vi "Sonicator Module (Main).vi"(7 "Name of Parent Panel":string="Main.vi", 9 "New Center Coords":T1={"Horizontal"=470, "Vertical"=200}, 10 "Config":variant, 11 "Main UI Message Queue":refnum<queue>) -> ()   [LabVIEW 2018, in "Sonicator Module.lvlib"]
doc: "This Continuous Measurement sample project is based on the Queued Message Handler template.\n\nThe Event Handling Loop generates messages based on user interface actions.\n\nThe Message Handling Loop processes messages generated by the Event Handling Loop, or by other messages. There are also Acquisition and Logging message handling loop subVIs, and a chart updating loop."
uses:
  Sonicator Module.lvlib
  support/Message Queue/Message Cluster.ctl
  <vilib>/Utility/miscctls.llb/LVPoint32TypeDef.ctl
  controls/UI State.ctl
  Feed Module/Controls/Sonicator Module Config Cluster.ctl
  Feed Module/Controls/Sonicator Module Settings Cluster.ctl
  Sonic Systems P100/Sonic Systems P100 Settings.ctl
  Feed Module/Controls/Sonicator Module State Cluster.ctl
  Pump Module Folder/Measure Instrument/State Enum.ctl
  Sequencing/Squence Update Cluster.ctl
  Measure Instrument/State Enum.ctl
  Feed Module/Controls/Sonicator Module Display.ctl
  support/Message Queue/Enqueue Message (Single).vi
  support/User Event - Stop/User Event - Stop.lvlib
  support/Message Queue/Message Queue.lvlib
  support/Support Library.lvlib
  Measure Instrument/Sonicator Module Engine.lvlib
  Sonicator Settings Dialog.vi
  support/Command Log VIs/Command Logging.lvlib
  Sonic Systems P100/Sonic Systems P100.lvlib
  Pump Module Folder/Measure Instrument/Pump Module Engine.lvlib
  Sequencing/Sequencing Library.lvlib
  Measure Instrument/Feed Module Engine.lvlib
  Report Generation/Report Generation.lvlib
panel:
  in  "Settings Button":bool
  out "Display Cluster":cluster{"User Name":string, "µm":dbl, "W":dbl} {"W" format="%#_5f"; "µm" format="%#_5f"}
  out "Ring":u16(ring)=2
  out "Original Width":u32
  out "Original Height":u32
  out "H/W":dbl
  out "ScanCode":i16
  out "Log File path":path
  out "Status":string
  in  "Exit":bool
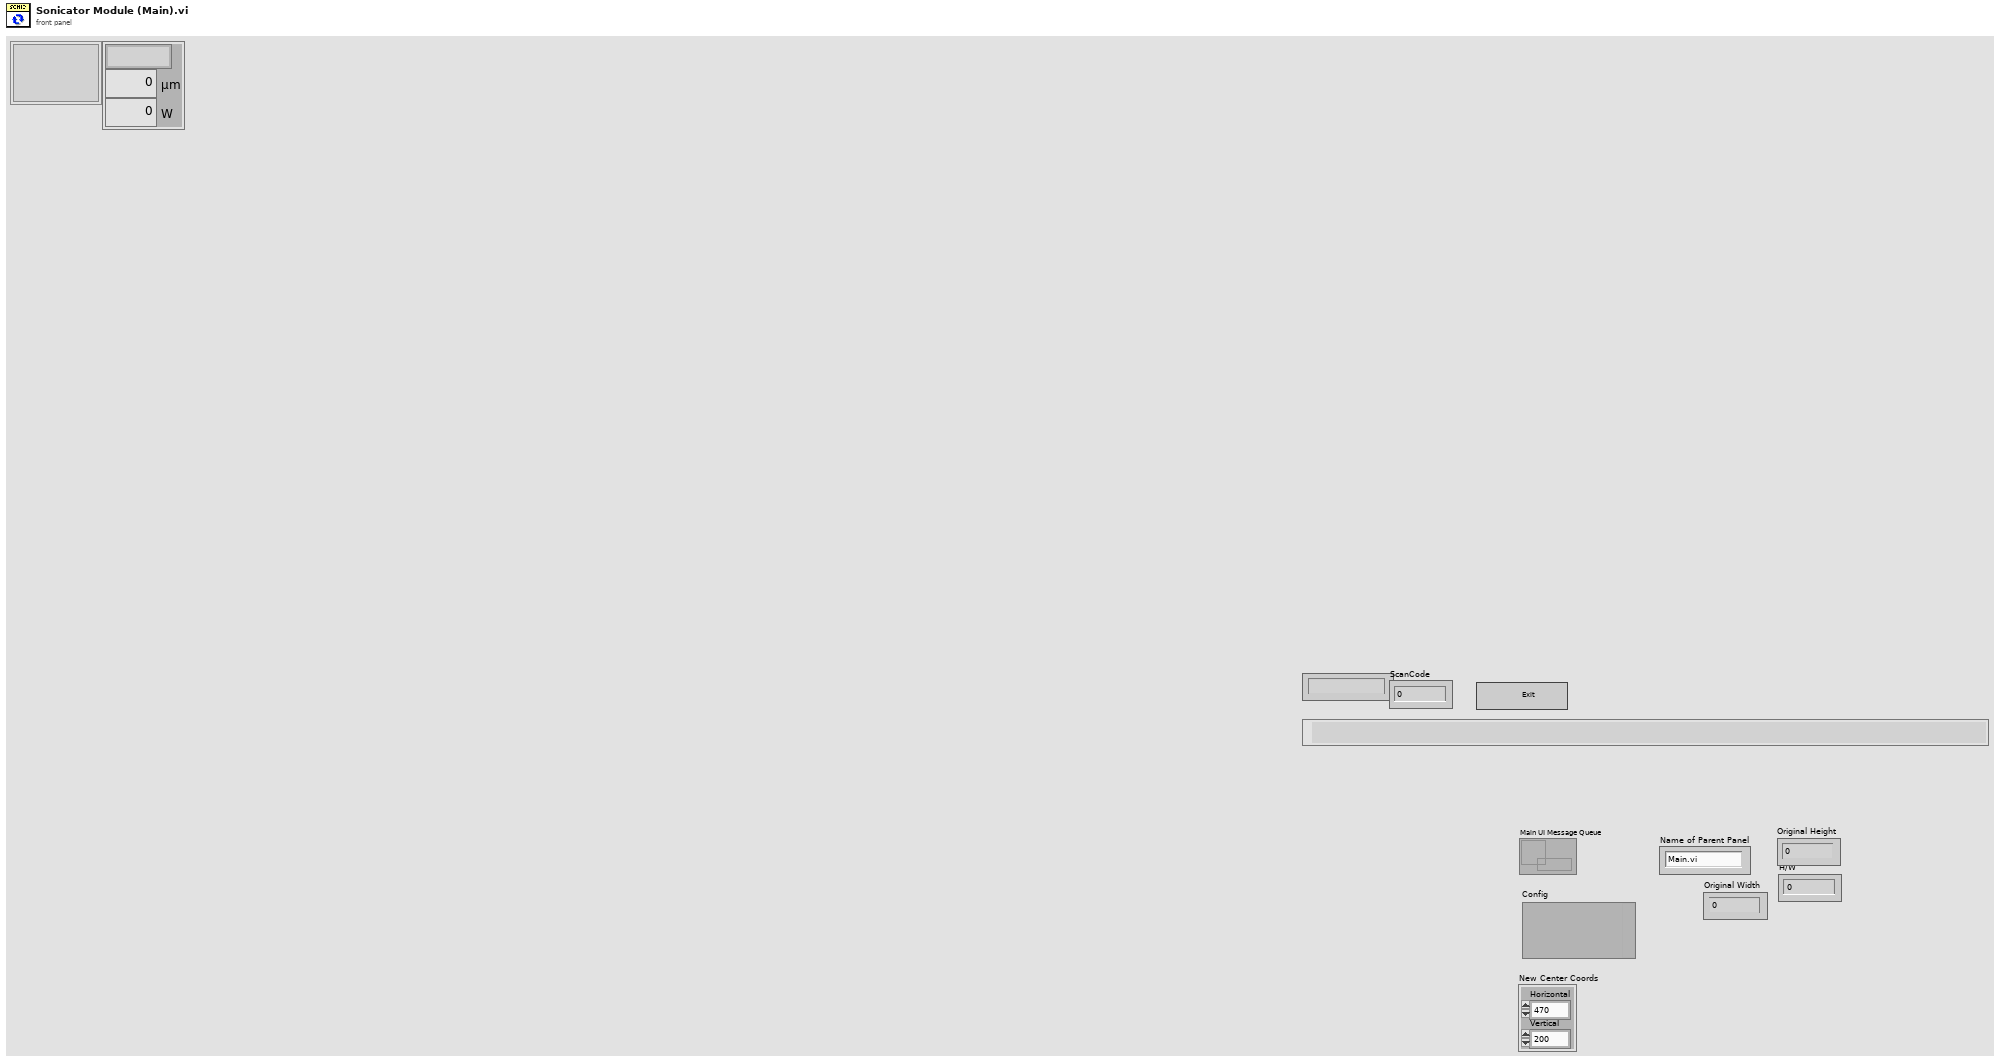
[diagram p1: front panel]
types:
  T1 = typedef "LVPoint32TypeDef.ctl" = cluster{"Horizontal":i32, "Vertical":i32}
  T2 = enum32{"Invalid", "Default", "Floating", "Floating/Auto-Hide", "Modal"}
  T3 = typedef "Sonicator Module.lvlib/Sonicator Module Config Cluster.ctl" = cluster{"GUID":string, "Drop Coords":T1, "Process Name":string, "User name":string, "Queue Name":string, "Settings":T4, "Load Count":i32}
  T4 = typedef "Sonicator Module.lvlib/Sonicator Module Settings Cluster.ctl" = cluster{"Cycle Period":dbl, "Sonicator Type":string, "SS P100 Settings":T5, "Setpoint (µm)":dbl, "Cutoff (W)":dbl}
  T5 = typedef "Sonic Systems P100.lvlib/Sonic Systems P100 Settings.ctl" = cluster{"VISA resource name":refnum<visa-resource-name>, "Simulated?":bool}
  T6 = typedef "UI State.ctl" = enum16{"Idle", "Acquiring and Logging", "Waiting for Exit", "Waiting for Exit (Acq Stopped)", "Waiting for Exit (Log Stopped)", "Waiting for Stop", "Waiting for Stop (Acq Stopped)", "Waiting for Stop (Log Stopped)"}
  T7 = typedef "Sonicator Module.lvlib/Sonicator Module State Cluster.ctl" = cluster{"State":T8, "Start Time":timestamp, "Current Time":timestamp, "Sonicator Module Config":T3, "Output Error":bool, "Log Started":bool, "First Iteration":bool, "Data":cluster{"Sonicator Amp Value":dbl, "Sonicator Power Value":dbl}, "Sonicator On?":enum16{"Off", "On", "Not Initialized", "Over Cutoff"}}
  T8 = typedef "Pump Module.lvlib/Pump Module Engine.lvlib/State Enum.ctl" = enum16{"Measuring", "Idle", "Paused"}
  T9 = typedef "LVPointTypeDef.ctl" = cluster{"Horizontal":i16, "Vertical":i16}
  T10 = typedef "Sonicator Module.lvlib/Sonicator Message Queues.ctl" = cluster{"Sonicator UI":refnum<queue>, "Sonicator Engine":refnum<queue>, "Sonicator Display":refnum<queue>}
  T11 = typedef "Sequencing Library.lvlib/Squence Update Cluster.ctl" = cluster{"Auto?":bool, "Manual Entry":dbl, "Setpoint":dbl}
  T12 = typedef "Feed Module.lvlib/Feed Module Engine.lvlib/State Enum.ctl" = enum16{"Measuring", "Idle", "Paused"}
  T13 = typedef "Sonicator Module.lvlib/Sonicator Module Display.ctl" = cluster{"Sonicator On?":enum16{"Off", "On", "Not Initialized", "Over Cutoff"}, "Sonicator Amp Value":dbl, "Sonicator Power Value":dbl, "Cycle Period":dbl}
  T14 = enum16{"Off", "On", "Not Initialized", "Over Cutoff"}
  T15 = typedef "LVRectTypeDef.ctl" = cluster{"Left":i16, "Top":i16, "Right":i16, "Bottom":i16}
  T16 = cluster{"Shift":bool, "Ctrl":bool, "Alt":bool, "Cmd":bool, "Opt":bool}
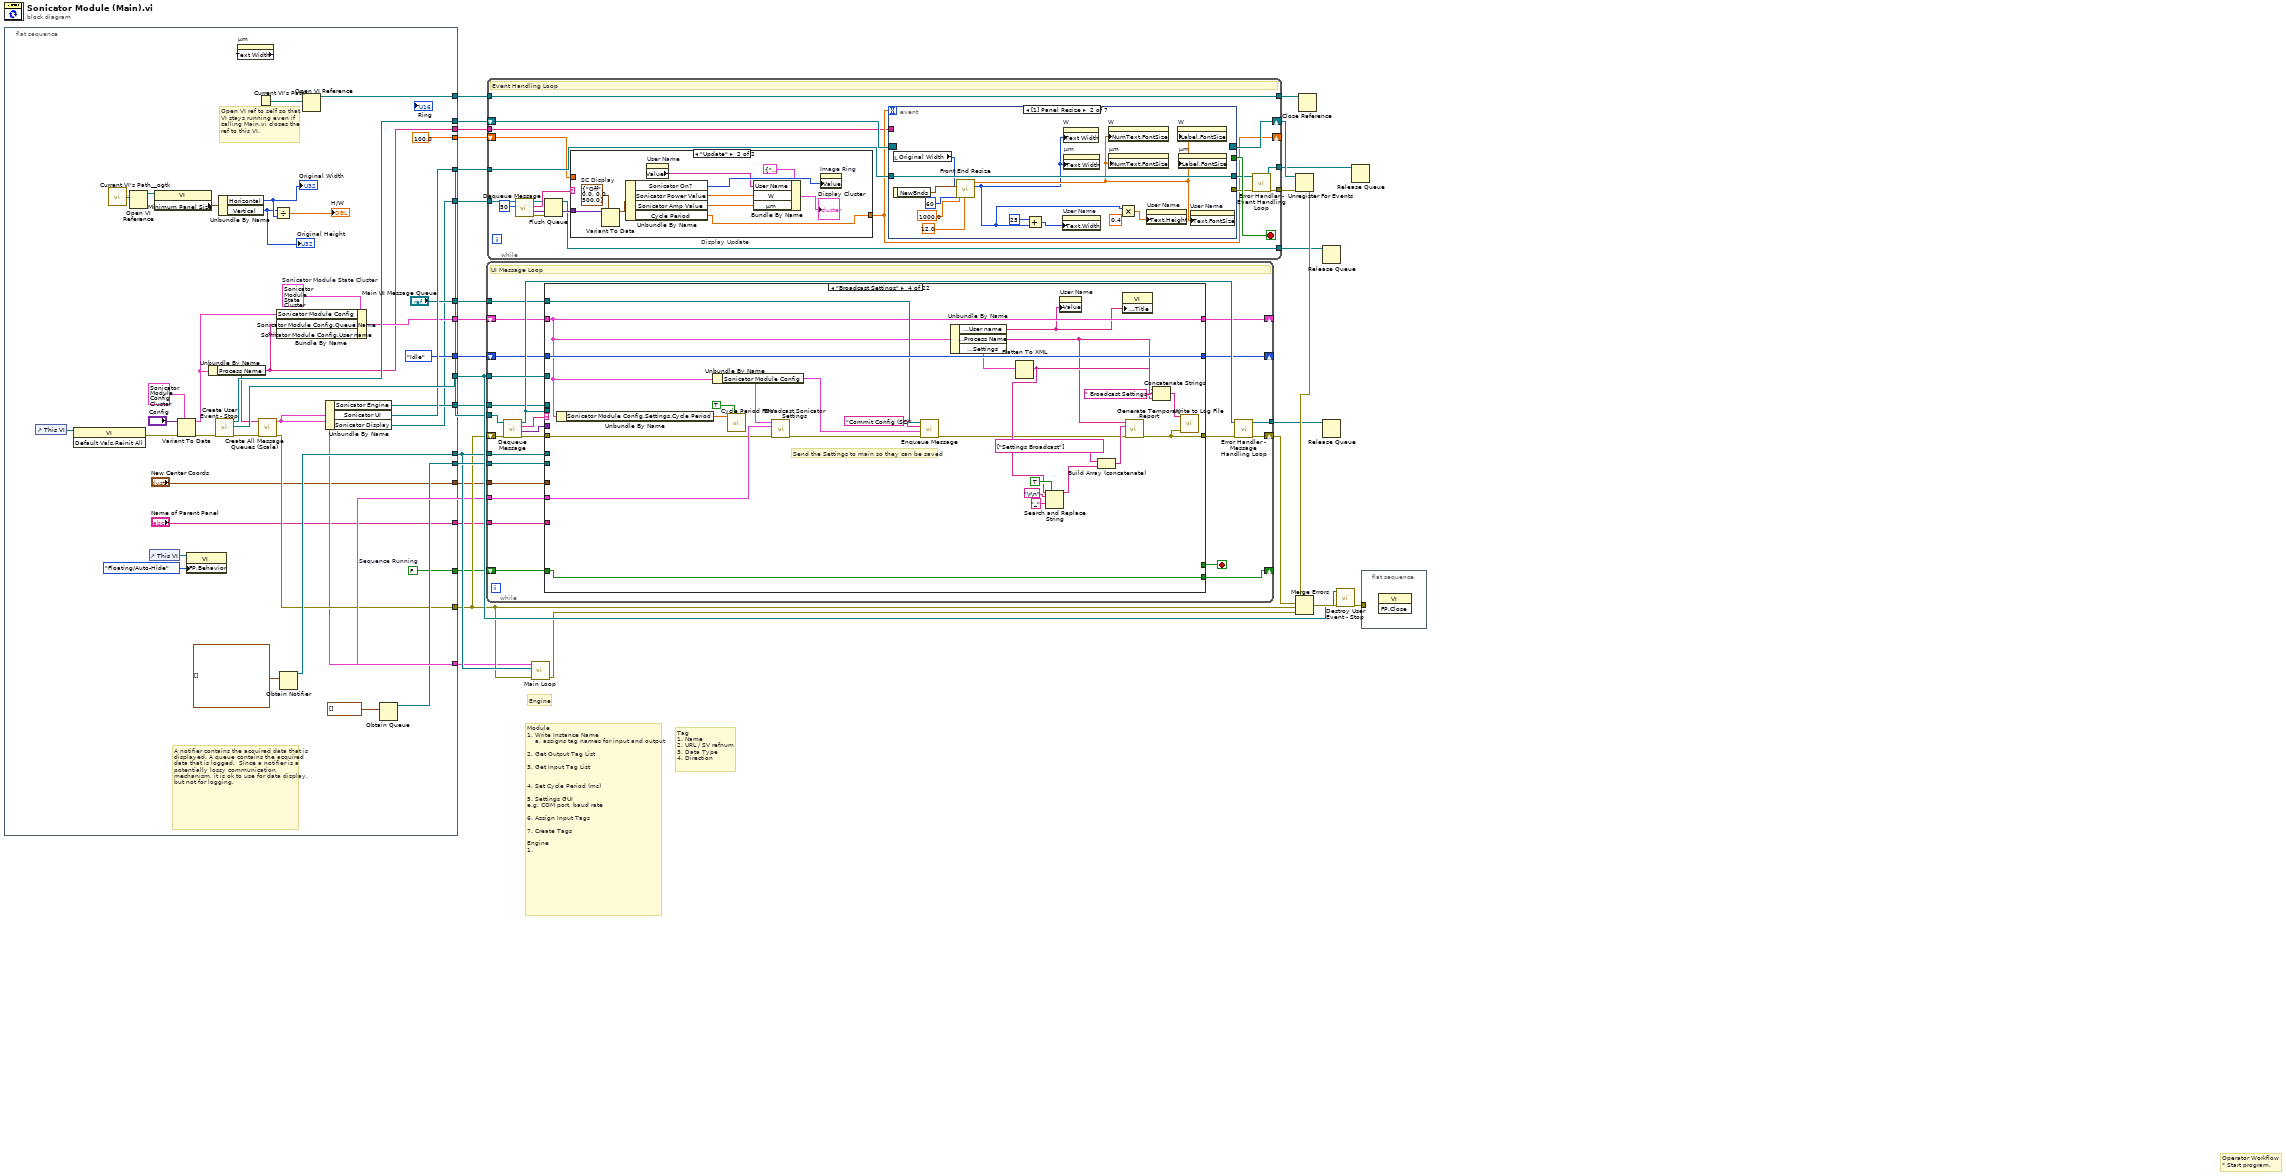
[diagram p0: block diagram]
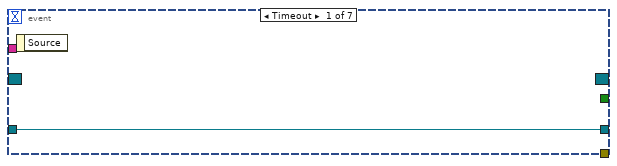
[diagram p3: hidden frame]
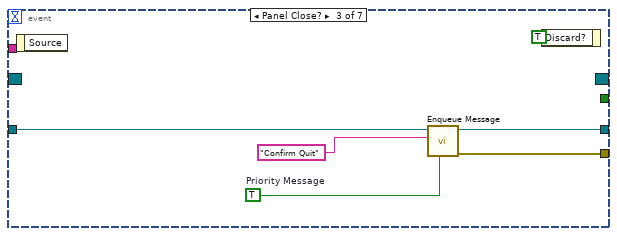
[diagram p4: hidden frame]
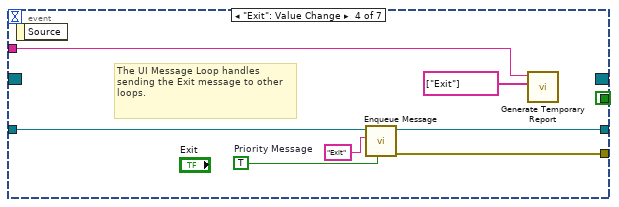
[diagram p5: hidden frame]
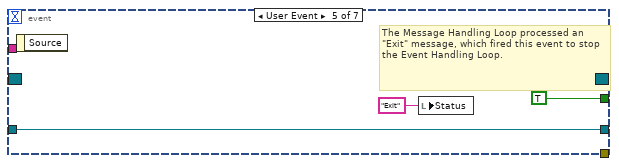
[diagram p6: hidden frame]
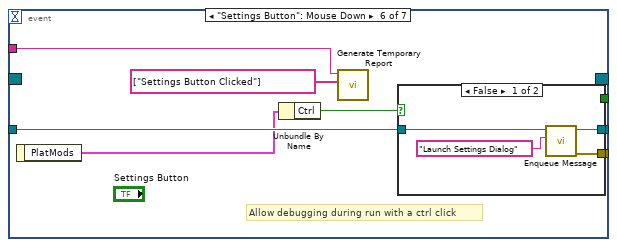
[diagram p7: hidden frame]
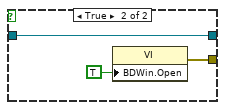
[diagram p8: hidden frame]
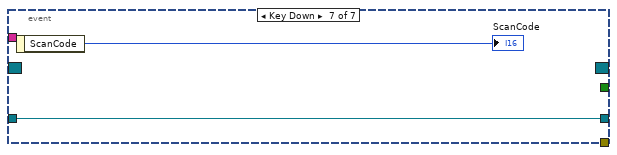
[diagram p9: hidden frame]
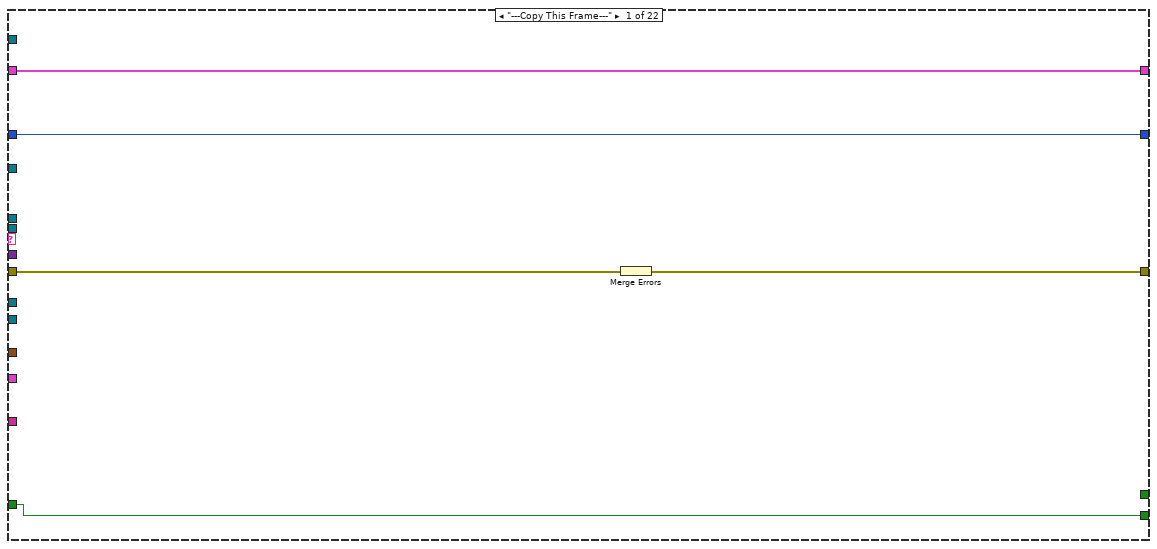
[diagram p10: hidden frame]
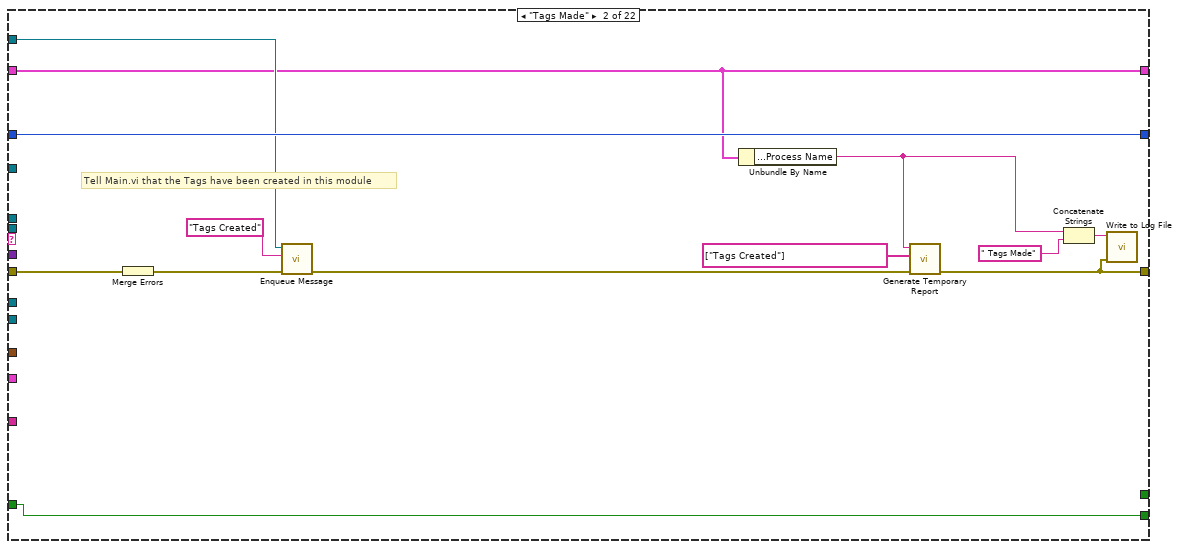
[diagram p11: hidden frame]
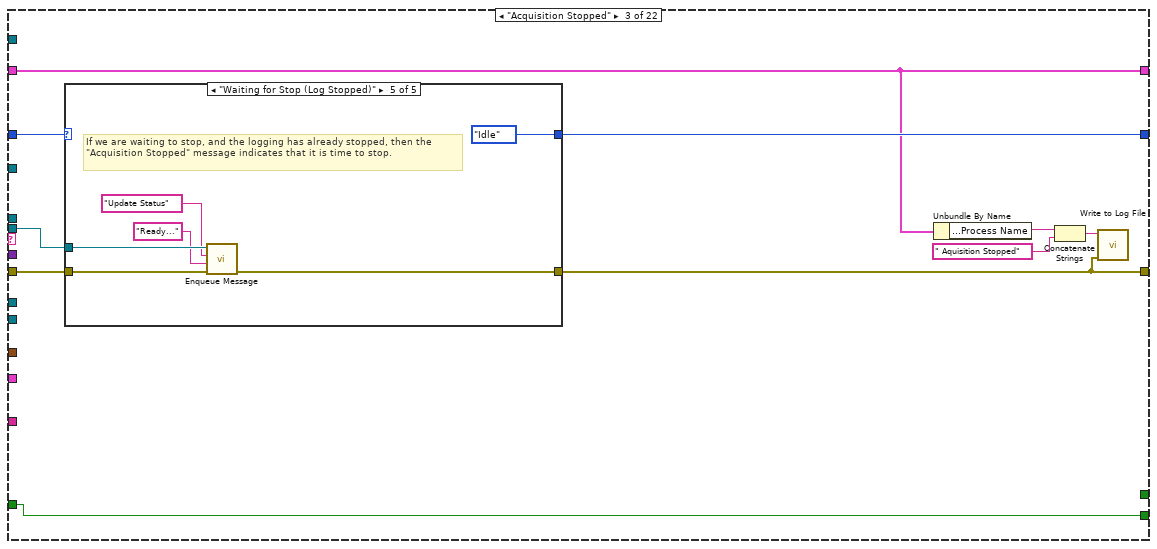
[diagram p12: hidden frame]
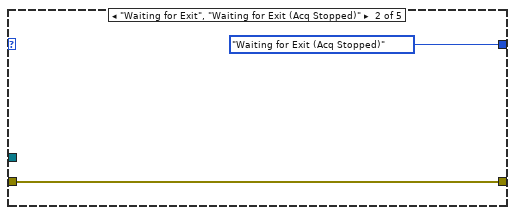
[diagram p14: hidden frame]
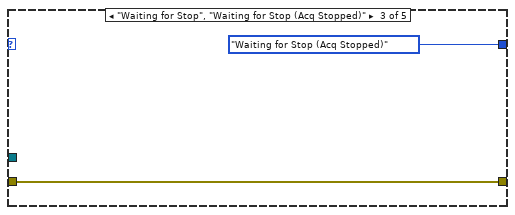
[diagram p15: hidden frame]
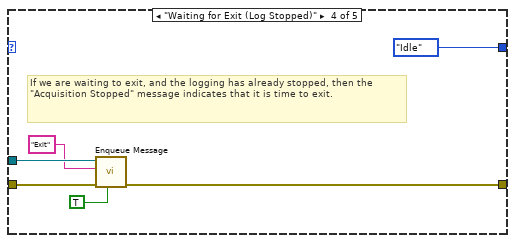
[diagram p16: hidden frame]
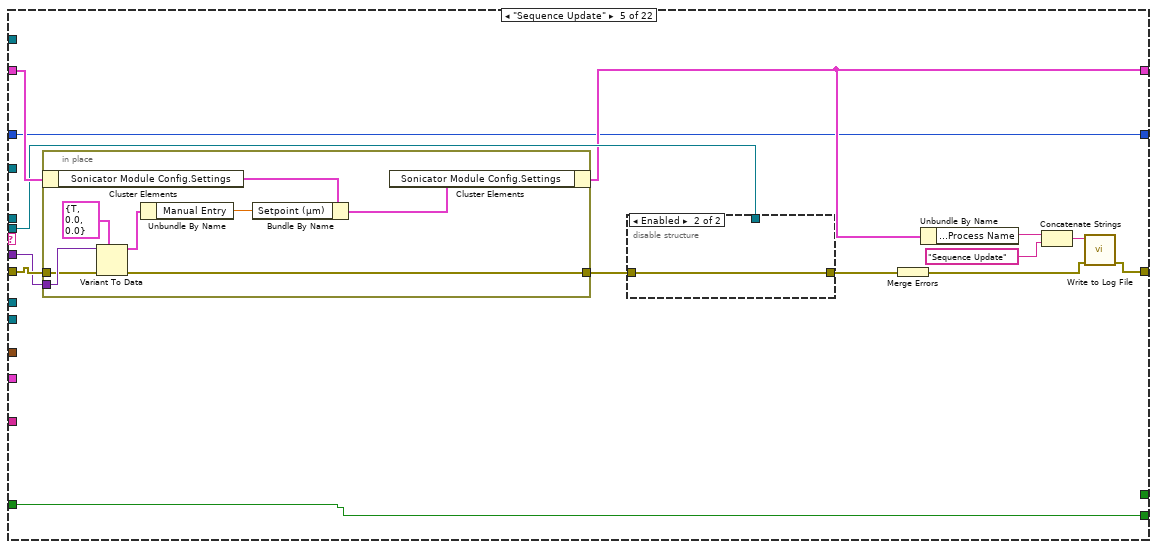
[diagram p17: hidden frame]
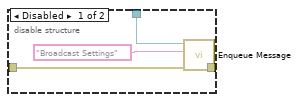
[diagram p18: hidden frame]
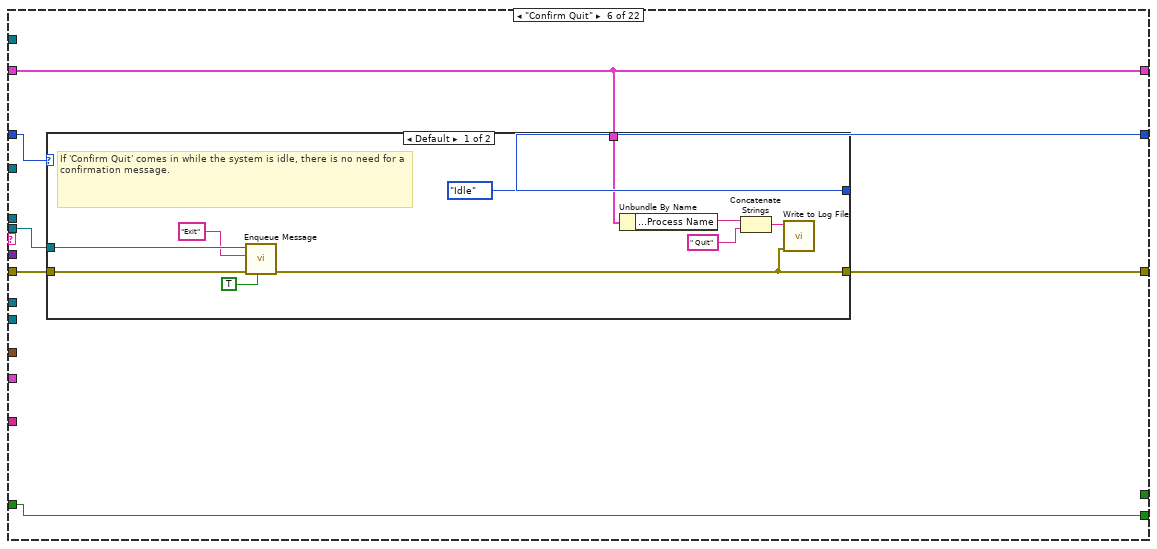
[diagram p19: hidden frame]
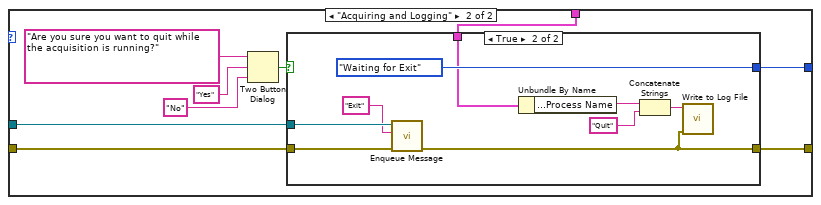
[diagram p20: hidden frame]
diagram:
  # "Engine"
  # "Operator Workflow\n* Start program."
  # "Module \n1. Write Instance Name\n    a. assigns tag names for input and output\n\n2. Get Output Tag List\n\n3. Get Input Tag List\n\n\n4. Set Cycle Period (ms)\n\n5. Settings GUI\ne.g. COM port, baud rate\n\n6. Assign Input Tags\n\n7. Create Tags\n\nEngine\n1."
  # "Tag\n1. Name\n2. URL / SV refnum\n3. Data Type\n4. Direction"
  n1 = flat-sequence {
    tunnel: [w66] -> w26
    tunnel: [w65] -> w25
    tunnel: [w64] -> w22
    tunnel: [UI_State."Idle" ("UI State")] -> w21
    tunnel: [w60] -> w20
    tunnel: [w59] -> w19
    tunnel: [w58] -> w17
    tunnel: [w57] -> w15
    tunnel: [w55] -> w14
    tunnel: ["Main UI Message Queue"] -> w13
    tunnel: [w50] -> w12
    tunnel: [w45] -> w11
    tunnel: [w44] -> w10
    tunnel: ["New Center Coords"] -> w9
    tunnel: ["Name of Parent Panel"] -> w8
    tunnel: [100.0 ("Cycle Period")] -> w6
    tunnel: [w37] -> w2
    tunnel: [w36] -> w1
    frame #0 {
      w37 = FALSE  # Sequence Running
      w51 = T7 {"State"=enum."Idle", "Start Time"=timestamp(0 s since 1904-01-01), "Current Time"=timestamp(0 s since 1904-01-01), "Sonicator Module Config"={"GUID"="PID1-Mettler Toledo Scale 1", "Drop Coords"={"Horizontal"=0, "Vertical"=0}, "Process Name"="PID1-Setpoint", "User name"="", "Queue Name"="", "Settings"={"Cycle Period"=500.0, "Sonicator Type"="", "SS P100 Settings"={"VISA resource name"="", "Simulated?"=FALSE}, "Setpoint (µm)"=0.0, "Cutoff (W)"=0.0}, "Load Count"=0}, "Output Error"=FALSE, "Log Started"=FALSE, "First Iteration"=FALSE, "Data"={"Sonicator Amp Value"=0.0, "Sonicator Power Value"=0.0}, "Sonicator On?"=enum."Off"}  # Sonicator Module State Cluster
      # "Open VI ref to self so that\nVI stays running even if\ncalling Main.vi closes the\nref to this VI."
      # "A notifier contains the acquired data that is displayed. A queue contains the acquired data that is logged.  Since a notifier is a potentially lossy communication mechanism, it is ok to use for data display, but not for logging."
      n2 = control-ref of="This VI"() -> (w48:refnum<vi>)
      n3 = invoke class="VI" method="Default Vals.Reinit All"(reference=w48) -> (error out=w41:errorcluster)  [unwired: 2 in, 2 out]
      n4 = call <userlib>:"Current VI's Path__ogtk.vi"() -> ("Current VI's Path (+ Relative)"=w34:path)  [unwired: 1 in]
      n5 = Open VI Reference(vi path=w34) -> (vi reference=w33:refnum<vi>)  [unwired: 5 in, 1 out]
      n6 = control-ref of="This VI"() -> (w39:refnum<vi>)
      n7 = property class="VI"(reference=w33) -> ("Minimum Panel Size"=w32:T9)  [unwired: 1 in, 2 out]
      n8 = Variant To Data(error in=w41, type=T3 {"GUID"="", "Drop Coords"={"Horizontal"=0, "Vertical"=0}, "Process Name"="", "User name"="", "Queue Name"="", "Settings"={"Cycle Period"=500.0, "Sonicator Type"="", "SS P100 Settings"={"VISA resource name"="", "Simulated?"=FALSE}, "Setpoint (µm)"=0.0, "Cutoff (W)"=0.0}, "Load Count"=0} ("Feed Module Config"), Variant="Config") -> (data=w49:T3, error out=w54:errorcluster)
      n9 = property class="VI"(reference=w39, "FP.Behavior"=T2."Floating/Auto-Hide" ("Front Panel Window:Behavior")) -> ()  [unwired: 1 in, 2 out]
      n10 = Unbundle By Name(w49) -> ("Process Name"=w36:string)
      n11 = call "Create User Event - Stop.vi"("error in (no error)"=w54) -> ("error out"=w46:errorcluster, "User Event - Stop"=w65:refnum<user-event>, "Stop Event Registration Refnum"=w66:refnum<event-registration>)  [unwired: 8 in]
      n12 = Unbundle By Name(w32) -> ("Horizontal"=w31:i16, "Vertical"=w30:i16)
      "Original Width" <- w31
      "Original Height" <- w30
      n13 = property on="µm" class="DigNum (strict)" props=["Text Width"]() -> ()  [unwired: 2 in, 3 out]
      n14 = Current VI's Path() -> (path=w56:path)
      n15 = call "Create All Message Queues (Scale).vi"("error in (no error)"=w46, "Process Name"=w36) -> ("error out"=w45:errorcluster, "Message Queues"=w44:T10)  [unwired: 8 in]
      n16 = Divide(x=w30, y=w31) -> (x/y=→"H/W":dbl)
      n17 = Bundle By Name(cluster=w51, "Sonicator Module Config"=w49, "Sonicator Module Config.Queue Name"=w36, "Sonicator Module Config.User name"=w36) -> (w55:T7)
      n18 = Obtain Notifier(notification data type=waveform(dbl)[] []) -> (notifier out=w58:refnum<notifier>)  [unwired: 3 in, 2 out]
      n19 = Open VI Reference(vi path=w56) -> (vi reference=w57:refnum<vi>)  [unwired: 5 in, 1 out]
      n20 = Unbundle By Name(w44) -> ("Sonicator Engine"=w60:refnum<queue>, "Sonicator UI"=w64:refnum<queue>, "Sonicator Display"=w50:refnum<queue>)
      n21 = Obtain Queue(element data type=waveform(dbl)[] []) -> (queue out=w59:refnum<queue>)  [unwired: 4 in, 2 out]
    }
  }
  n22 = while {
    tunnel: w22 -> [w85]
    tunnel: w25 -> [w89]
    shift-right: [w81] -> w29
    shift-left: w11 -> [w88]
    shift-right: [w72] -> _
    shift-left: w14 -> [w74]
    tunnel: w17 -> [w84]
    tunnel: w19 -> [w83]
    shift-right: [w78] -> _
    shift-left: w21 -> [w79]
    tunnel: w20 -> [w77]
    tunnel: w10 -> [w76]
    tunnel: w13 -> [w73]
    tunnel: w9 -> [w71]
    tunnel: w8 -> [w70]
    tunnel: [w69] -> w3
    shift-right: [w67] -> _
    shift-left: w2 -> [w68]
    stop <- w90 stop-if-true
    # "UI Message Loop"
    n23 = call "Dequeue Message.vi"("error in (no error)"=w88, "Message Queue"=w85) -> ("error out"=w75:errorcluster, "Message Data"=w86:variant, "Message"=w87:string, "dup Message Queue"=w80:refnum<queue>)  [unwired: 6 in]
    n24 = case "Message Cases" shown="\"Broadcast Settings\"" w87 {
      selector: w87 -> [_ _ _ _ _ _ _ _ _ _ _ _ _ _ _ _ _ _ _ _ _ w489]
      tunnel: w80 -> [_ _ w115 _ w165 w194 _ w248 w263 w288 _ w331 _ w357 _ w398 w402 _ _ w475 _ _]
      tunnel: w75 -> [w95 w108 w116 w157 w169 w193 w229 w243 w267 w287 w314 w327 w347 w358 w384 w397 w403 w430 w442 w470 w485 _]
      tunnel: [w94 w96 w111 w138 w168 w192 w230 w235 w254 w268 w314 w318 w346 w353 w387 w393 w406 w426 w444 w458 w486 w488] -> w82
      tunnel: [_ _ _ _ _ _ _ _ _ TRUE _ _ _ _ _ _ _ _ _ _ _ _] -> w90
      tunnel: w86 -> [_ _ _ _ w166 _ w232 _ w266 w277 _ _ _ _ w385 _ _ _ _ _ w484 _]
      tunnel: w89 -> [_ _ _ _ _ _ _ _ _ w298 _ _ _ _ _ _ _ _ _ _ _ _]
      tunnel: w74 -> [w92 w101 w110 w150 w167 w190 w227 w239 w253 w273 w311 w317 w342 w352 w390 w392 w409 w431 w443 w463 w479 w494]
      tunnel: w84 -> [_ _ _ _ _ _ _ _ _ w296 _ _ _ _ _ _ _ _ _ _ _ _]
      tunnel: w83 -> [_ _ _ _ _ _ _ _ _ w292 _ _ _ _ _ _ _ _ _ _ _ _]
      tunnel: w79 -> [w93 w107 w118 w161 w163 w195 w228 w244 w258 w285 _ _ w348 w360 w389 _ _ _ _ w471 w480 w498]
      tunnel: [w93 w107 w117 w161 w163 w191 w228 w245 w258 w284 UI_State."Idle" ("UI State") UI_State."Idle" ("UI State") w348 w359 w389 UI_State."Acquiring and Logging" ("UI State") UI_State."Acquiring and Logging" ("UI State") UI_State."Acquiring and Logging" ("UI State") UI_State."Acquiring and Logging" ("UI State") w472 w480 w498] -> w78
      tunnel: w77 -> [_ _ _ _ _ _ _ _ _ w291 _ _ _ _ _ _ _ w434 w451 w469 _ _]
      tunnel: w76 -> [_ _ _ w160 _ _ _ _ _ _ _ _ w339 _ _ _ _ _ _ _ _ _]
      tunnel: w73 -> [_ w104 _ w154 _ _ _ _ _ w276 _ _ _ _ _ _ _ _ _ _ _ _]
      tunnel: [w92 w101 w110 w150 w164 w190 w227 w239 w253 w273 w311 w317 w341 w352 w390 w392 w408 w431 w443 w463 w479 w494] -> w72
      tunnel: w71 -> [_ _ _ _ _ _ _ _ _ _ _ w325 _ _ _ _ _ _ _ _ _ _]
      tunnel: w70 -> [_ _ _ _ _ _ _ _ _ _ _ w324 _ _ _ _ _ _ _ _ _ _]
      tunnel: w68 -> [w91 w100 w109 w148 w162 w189 w226 w238 w251 w272 w310 w321 w338 w351 w381 w391 w404 w429 w441 w462 w478 w487]
      tunnel: [w91 w100 w109 w148 w162 w189 w226 w238 w251 w272 w310 w321 w338 w351 w381 w391 w405 w429 w441 w462 w478 w487] -> w67
      frame "---Copy This Frame---" {
        # "Duplicate this frame when creating new messages.  Change this comment in the duplicated frame to describe this message."
        n25 = Merge Errors(w95) -> (w94:errorcluster)
      }
      frame "Tags Made" {
        # "Tell Main.vi that the Tags have been created in this module"
        # "Duplicate this frame when creating new messages.  Change this comment in the duplicated frame to describe this message."
        n26 = Merge Errors(w108) -> (w105:errorcluster)
        n27 = call-poly "Enqueue Message.vi"("error in (no error)"=w105, "Message"="Tags Created", "Message Queue"=w104) -> ("error out"=w97:errorcluster)  [unwired: 7 in, 1 out]
        n28 = Unbundle By Name(w101) -> ("Sonicator Module Config.Process Name"=w98:string)
        n29 = call "Generate Temporary Report.vi"("error in (no error)"=w97, "Line of Events"=string[] ["Tags Created"], "Module Name"=w98) -> ("error out"=w96:errorcluster)  [unwired: 8 in]
        n30 = Concatenate Strings(w98, " Tags Made" ("text")) -> (w102:string)
        n31 = call "Write to Log File.vi"("error in"=w96, "text"=w102) -> ()  [unwired: 9 in, 1 out]
      }
      frame "Acquisition Stopped" {
        # "Logic for determining what action to take when the acquisition has stopped."
        n32 = case shown="\"Waiting for Stop (Log Stopped)\"" w118 {
          selector: w118 -> [w120 _ _ _ _]
          tunnel: [w120 UI_State."Waiting for Exit (Acq Stopped)" ("UI State") UI_State."Waiting for Stop (Acq Stopped)" ("UI State") UI_State."Idle" ("UI State") UI_State."Idle" ("UI State")] -> w117
          tunnel: w116 -> [w119 w121 w123 w129 w135]
          tunnel: [w119 w121 w123 w128 w134] -> w111
          tunnel: w115 -> [_ _ _ w127 w133]
          frame Default {
          }
          frame "Waiting for Exit", "Waiting for Exit (Acq Stopped)" {
          }
          frame "Waiting for Stop", "Waiting for Stop (Acq Stopped)" {
          }
          frame "Waiting for Exit (Log Stopped)" {
            # "If we are waiting to exit, and the logging has already stopped, then the \"Acquisition Stopped\" message indicates that it is time to exit."
            n33 = call-poly "Enqueue Message.vi"("Priority Message? (F)"=TRUE, "error in (no error)"=w129, "Message"="Exit", "Message Queue"=w127) -> ("error out"=w128:errorcluster)  [unwired: 6 in, 1 out]
          }
          frame "Waiting for Stop (Log Stopped)" {
            # "If we are waiting to stop, and the logging has already stopped, then the \"Acquisition Stopped\" message indicates that it is time to stop."
            n34 = call-poly "Enqueue Message.vi"("error in (no error)"=w135, "Message Data"="Ready..." ("Message"), "Message"="Update Status", "Message Queue"=w133) -> ("error out"=w134:errorcluster)  [unwired: 6 in, 1 out]
          }
        }
        n35 = Unbundle By Name(w110) -> ("Sonicator Module Config.Process Name"=w114:string)
        n36 = Concatenate Strings(w114, " Aquisition Stopped" ("text")) -> (w112:string)
        n37 = call "Write to Log File.vi"("error in"=w111, "text"=w112) -> ()  [unwired: 9 in, 1 out]
      }
      frame "Broadcast Settings" {
        # "Send the Settings to main so they can be saved"
        # "Send the 'Update Settings' message to the Logging and Acquisition message loops."
        n38 = Unbundle By Name(w150) -> ("Sonicator Module Config.Settings.Cycle Period"=w158:dbl)
        n39 = Unbundle By Name(w150) -> ("Sonicator Module Config"=w153:T3)
        n40 = call "Cycle Period FGV.vi"("Write"=TRUE, "Cycle Period In (ms)"=w158) -> ()  [unwired: 8 in, 2 out]
        n41 = call "Broadcast Sonicator Settings.vi"("error in (no error)"=w157, "Message Queues"=w160, "Scale Module Config"=w153) -> ("error out"=w155:errorcluster)  [unwired: 8 in]
        n42 = call-poly "Enqueue Message.vi"("error in (no error)"=w155, "Message Data"=w153, "Message"="Commit Config (SC)", "Message Queue"=w154) -> ("error out"=w139:errorcluster)  [unwired: 6 in, 1 out]
        n43 = Unbundle By Name(w150) -> ("Sonicator Module Config.User name"=w137:string, "Sonicator Module Config.Process Name"=w140:string, "Sonicator Module Config.Settings"=w149:T4)
        n44 = Flatten To XML(anything=w149) -> (xml string=w142:string)
        n45 = Search and Replace String(replace all?=TRUE ("replace all? (F)"), input string=w142, search string="\r\n", replace string="_" ("replace string (\"\")")) -> (result string=w143:string)  [unwired: 4 in, 3 out]
        n46 = property on="User Name" class="Str"("Value"=w137) -> ()  [unwired: 2 in, 2 out]
        n47 = Build Array (concatenate)(string[] ["Settings Broadcast"] ("Line of Events"), w143) -> (w141:string[])
        n48 = property class="VI"("Front Panel.Title"=w137) -> ()  [unwired: 2 in, 2 out]
        n49 = call "Generate Temporary Report.vi"("error in (no error)"=w139, "Line of Events"=w141, "Module Name"=w140) -> ("error out"=w138:errorcluster)  [unwired: 8 in]
        n50 = Concatenate Strings(w140, " Broadcast Settings: " ("text"), w142) -> (w151:string)
        n51 = call "Write to Log File.vi"("error in"=w138, "text"=w151) -> ()  [unwired: 9 in, 1 out]
      }
      frame "Sequence Update" {
        n52 = in-place {
          in-place-border: w166 -> [w185]
          in-place-border: w169 -> [w184]
          in-place-border: [w183] -> w174
          n53 = in-place-cluster #1(w167) -> ("Sonicator Module Config.Settings"=w181:T4)
          n54 = Variant To Data(error in=w184, type=T11 {"Auto?"=TRUE, "Manual Entry"=0.0, "Setpoint"=0.0} ("Cluster"), Variant=w185) -> (data=w187:T11, error out=w183:errorcluster)
          n55 = Unbundle By Name(w187) -> ("Manual Entry"=w186:dbl)
          n56 = Bundle By Name(cluster=w181, "Setpoint (µm)"=w186) -> (w182:T4)
          n57 = in-place-cluster #1("Sonicator Module Config.Settings"=w182) -> (w164:T7)
        }
        n58 = disable-structure shown="Enabled" {
          disable-tunnel: [w179 w180] -> w175
          disable-tunnel: w165 -> [w177 _]
          disable-tunnel: w174 -> [w176 w180]
          frame Disabled {
            n59 = call-poly "Enqueue Message.vi"("error in (no error)"=w176, "Message"="Broadcast Settings", "Message Queue"=w177) -> ("error out"=w179:errorcluster)  [unwired: 7 in, 1 out]
          }
          frame Enabled {
          }
        }
        n60 = Merge Errors(w175) -> (w171:errorcluster)
        n61 = Unbundle By Name(w164) -> ("Sonicator Module Config.Process Name"=w173:string)
        n62 = Concatenate Strings(w173, "Sequence Update" ("text")) -> (w170:string)
        n63 = call "Write to Log File.vi"("error in"=w171, "text"=w170) -> ("error out"=w168:errorcluster)  [unwired: 9 in]
      }
      frame "Confirm Quit" {
        # "Confirm Quit - Message that can confirm whether or not the user wants to exit the application."
        n64 = case shown="Default" w195 {
          tunnel: w194 -> [w204 w211]
          tunnel: w193 -> [w203 w209]
          tunnel: [w197 w208] -> w192
          tunnel: [UI_State."Idle" ("UI State") w207] -> w191
          tunnel: w190 -> [w196 w206]
          frame Default {
            # "If 'Confirm Quit' comes in while the system is idle, there is no need for a confirmation message."
            n65 = call-poly "Enqueue Message.vi"("Priority Message? (F)"=TRUE, "error in (no error)"=w203, "Message"="Exit", "Message Queue"=w204) -> ("error out"=w197:errorcluster)  [unwired: 6 in, 1 out]
            n66 = Unbundle By Name(w196) -> ("Sonicator Module Config.Process Name"=w200:string)
            n67 = Concatenate Strings(w200, " Quit" ("text")) -> (w198:string)
            n68 = call "Write to Log File.vi"("error in"=w197, "text"=w198) -> ()  [unwired: 9 in, 1 out]
          }
          frame "Acquiring and Logging" {
            n69 = Two Button Dialog(message="Are you sure you want to quit while the acquisition is running?" ("Confirm Quit Message"), 1:"No" ("No"), 2:"Yes" ("Yes")) -> (T button?=w210:bool)
            n70 = case shown="True" w210 {
              tunnel: w211 -> [_ w225]
              tunnel: w209 -> [w215 w224]
              tunnel: [w215 w218] -> w208
              tunnel: [UI_State."Acquiring and Logging" ("UI State") UI_State."Waiting for Exit" ("UI State")] -> w207
              tunnel: w206 -> [_ w217]
              frame False {
                # "User did not want to quit."
              }
              frame True {
                n71 = call-poly "Enqueue Message.vi"("error in (no error)"=w224, "Message"="Exit", "Message Queue"=w225) -> ("error out"=w218:errorcluster)  [unwired: 7 in, 1 out]
                n72 = Unbundle By Name(w217) -> ("Sonicator Module Config.Process Name"=w221:string)
                n73 = Concatenate Strings(w221, "Quit" ("text")) -> (w219:string)
                n74 = call "Write to Log File.vi"("error in"=w218, "text"=w219) -> ()  [unwired: 9 in, 1 out]
              }
            }
          }
        }
      }
      frame "Display Log File Path" {
        n75 = Variant To Data(error in=w229, type=path "", Variant=w232) -> (data=→"Log File path":path, error out=w230:errorcluster)
      }
      frame "E-Stop" {
        # "E-Stop has no effect on the scale"
        # "Message Acquisition and Logging loops to stop"
        # "Stop the pumps."
        n76 = call-poly "Enqueue Message.vi"("error in (no error)"=w243, "Message Data"="Ready..." ("Ready..."), "Message"="Update Status", "Message Queue"=w248) -> ("error out"=w242:errorcluster)  [unwired: 6 in, 1 out]
        n77 = case shown="\"Waiting for Exit\"" w244 {
          selector: w244 -> [_ w250]
          tunnel: [UI_State."Waiting for Stop" ("UI State") w250] -> w245
          frame Default {
          }
          frame "Waiting for Exit" {
          }
        }
        n78 = Merge Errors(w242) -> (w236:errorcluster)
        n79 = Unbundle By Name(w239) -> ("Sonicator Module Config.Process Name"=w234:string)
        n80 = call "Generate Temporary Report.vi"("error in (no error)"=w236, "Line of Events"=string[] ["E-STOP"], "Module Name"=w234) -> ("error out"=w235:errorcluster)  [unwired: 8 in]
        n81 = Concatenate Strings(w234, " E-STOP" ("text")) -> (w240:string)
        n82 = call "Write to Log File.vi"("error in"=w235, "text"=w240) -> ()  [unwired: 9 in, 1 out]
      }
      frame "Error" {
        # "Error - Check the error message data and respond accordingly. This message is sent by the \"Error Handler\" VIs at the end of each loop in this application."
        n83 = Variant To Data(error in=w267, type=errorcluster {"status"=FALSE, "code"=0, "source"=""} ("error out"), Variant=w266) -> (data=w264:errorcluster, error out=w260:errorcluster)
        n84 = call <vilib>:"General Error Handler.vi"("error in (no error)"=w264) -> ("message"=w252:string)  [unwired: 10 in, 4 out]
        n85 = call-poly "Enqueue Message.vi"("Priority Message? (F)"=TRUE, "Message"="Exit", "Message Queue"=w263) -> ("error out"=w259:errorcluster)  [unwired: 7 in, 1 out]
        n86 = Merge Errors(w259, w260) -> (w254:errorcluster)
        n87 = Unbundle By Name(w253) -> ("Sonicator Module Config.Process Name"=w257:string)
        n88 = Concatenate Strings(w257, " Error: " ("text"), w252) -> (w255:string)
        n89 = call "Write to Log File.vi"("error in"=w254, "text"=w255) -> ()  [unwired: 9 in, 1 out]
      }
      frame "Exit" {
        w280 = TRUE  # Delete Module?
        # "Don't check the error outs. The acquisition and logging queues may have already been released."
        # "Close references owned by the Main VI."
        # "Stop the VI"
        # "Exit - Fire the User Event to stop the Event Handling Loop.  Also send Exit messages to the Acquisition and Logging loops."
        n90 = call "Fire User Event - Stop.vi"("User Event - Stop"=w298) -> ("error out"=w297:errorcluster)  [unwired: 10 in]
        n91 = Build Array(w291) -> (w290:refnum<queue>[])
        n92 = for {
          tunnel: w290 -> [w307] mode=indexing
          n93 = call-poly "Enqueue Message.vi"("Message"="Stop", "Message Queue"=w307) -> ("dup Message Queue"=w308:refnum<queue>)  [unwired: 8 in, 1 out]
          n94 = call-poly "Enqueue Message.vi"("Message"="Exit", "Message Queue"=w308) -> ()  [unwired: 8 in, 2 out]
        }
        n95 = Variant To Data(type=w280, Variant=w277) -> (data=w279:bool, error out=w281:errorcluster)  [unwired: 1 in]
        n96 = call-poly "Enqueue Message.vi"("error in (no error)"=w287, "Message Data"="Ready..." ("Ready..."), "Message"="Update Status", "Message Queue"=w288) -> ("error out"=w286:errorcluster, "dup Message Queue"=w283:refnum<queue>)  [unwired: 6 in]
        n97 = Select(t=w280, s=w281, f=w279) -> (s? t:f=w278:bool)
        n98 = case "Don't enqueue Delete Module if opening campaign because it\nwill already have been deleted and new config loaded and we create\na race condition." shown="True" w278 {
          tunnel: w276 -> [_ w302]
          tunnel: w273 -> [_ w301]
          frame False {
          }
          frame True {
            n99 = Unbundle By Name(w301) -> ("Sonicator Module Config.GUID"=w300:string)
            n100 = call-poly "Enqueue Message.vi"("Message Data"=w300, "Message"="Delete Module", "Message Queue"=w302) -> ()  [unwired: 7 in, 2 out]
          }
        }
        n101 = Release Queue(queue=w283, error in (no error)=w286) -> (error out=w295:errorcluster)  [unwired: 1 in, 2 out]
        n102 = Release Notifier(notifier=w296, error in (no error)=w295) -> (error out=w294:errorcluster)  [unwired: 1 in, 2 out]
        n103 = Release Queue(queue=w292, error in (no error)=w294) -> (error out=w293:errorcluster)  [unwired: 1 in, 2 out]
        n104 = Merge Errors(w297, w293) -> (w269:errorcluster)
        n105 = Unbundle By Name(w273) -> ("Sonicator Module Config.Process Name"=w270:string)
        n106 = case shown="Default" w285 {
          selector: w285 -> [_ w305]
          tunnel: [UI_State."Waiting for Stop" ("UI State") w305] -> w284
          frame Default {
          }
          frame "Waiting for Exit" {
          }
        }
        n107 = Concatenate Strings(w270, " Exit" ("text")) -> (w274:string)
        n108 = call "Generate Temporary Report.vi"("error in (no error)"=w269, "Line of Events"=string[] ["Exited"], "Module Name"=w270) -> ("error out"=w268:errorcluster)  [unwired: 8 in]
        n109 = call "Write to Log File.vi"("error in"=w268, "text"=w274) -> ()  [unwired: 9 in, 1 out]
      }
      frame "Init UI Refs" {
        # "Init UI Refs - Store control references for UI controls.  Also enable/disable controls appropriately."
        n110 = property class="VI"("Front Panel.Closeable"=TRUE ("Front Panel Window:Closeable")) -> ()  [unwired: 2 in, 2 out]
      }
      frame "Initialize" {
        # "Initialize - Get configuration settings, then message the UI to initialize, and broadcast the settings to the other message loops."
        n111 = Unbundle By Name(w317) -> ("Sonicator Module Config.Process Name"=w316:string)
        n112 = call-poly "Enqueue Message.vi"("error in (no error)"=w327, "Message"="Init UI Refs", "Message Queue"=w331) -> ("error out"=w329:errorcluster, "dup Message Queue"=w330:refnum<queue>)  [unwired: 7 in]
        n113 = property class="VI" props=["FP.State"]() -> (reference out=w326:refnum<vi>)  [unwired: 2 in, 2 out]
        n114 = call "Make Child and Move.vi"("Process Name"=w316, "Name of Parent Panel"=w324, "New Center Coords"=w325, "VI in"=w326) -> ()  [unwired: 8 in]
        n115 = call-poly "Enqueue Message.vi"("error in (no error)"=w329, "Message"="Broadcast Settings", "Message Queue"=w330) -> ("error out"=w337:errorcluster, "dup Message Queue"=w336:refnum<queue>)  [unwired: 7 in]
        n116 = call-poly "Enqueue Message.vi"("error in (no error)"=w337, "Message Data"="Ready..." ("Ready..."), "Message"="Update Status", "Message Queue"=w336) -> ("error out"=w319:errorcluster)  [unwired: 6 in, 1 out]
        n117 = Unbundle By Name(w317) -> ("Sonicator Module Config.Process Name"=w315:string)
        n118 = call "Generate Temporary Report.vi"("error in (no error)"=w319, "Line of Events"=string[] ["Initialize"], "Module Name"=w315) -> ("error out"=w318:errorcluster)  [unwired: 8 in]
        n119 = Concatenate Strings(w315, " Initialize" ("text")) -> (w322:string)
        n120 = call "Write to Log File.vi"("error in"=w318, "text"=w322) -> ()  [unwired: 9 in, 1 out]
      }
      frame "Launch Settings Dialog" {
        # "Launch the Settings Dialog when the user clicks the 'Settings' button."
        n121 = in-place {
          n122 = in-place-cluster #2(w342) -> ("Sonicator Module Config.Load Count"=w349:i32)
          n123 = Increment(x=w349) -> (x+1=w350:i32)
          n124 = in-place-cluster #2("Sonicator Module Config.Load Count"=w350) -> (w340:T7)
        }
        n125 = call-by-ref "?"("error in (no error)"=w347, "Message Queues"=w339, "Sonicator Module State Cluster"=w340) -> ("error out"=w346:errorcluster, "Sonicator Module State Cluster"=w341:T7)  [unwired: 7 in, 4 out]
        n126 = Unbundle By Name(w341) -> ("Sonicator Module Config.Process Name"=w345:string)
        n127 = Concatenate Strings(w345, " Setting Dialog Launched" ("text")) -> (w343:string)
        n128 = call "Write to Log File.vi"("error in"=w346, "text"=w343) -> ()  [unwired: 9 in, 1 out]
      }
      frame "Logging Stopped" {
        # "Logic for determining what action to take when the logging has stopped."
        n129 = case shown="\"Waiting for Exit (Acq Stopped)\"" w360 {
          selector: w360 -> [w362 _ _ _ _]
          tunnel: [w362 UI_State."Waiting for Exit (Log Stopped)" ("UI State") UI_State."Waiting for Stop (Log Stopped)" ("UI State") UI_State."Idle" ("UI State") UI_State."Idle" ("UI State")] -> w359
          tunnel: w358 -> [w361 w363 w365 w371 w377]
          tunnel: [w361 w363 w365 w370 w376] -> w353
          tunnel: w357 -> [_ _ _ w369 w375]
          frame Default {
          }
          frame "Waiting for Exit", "Waiting for Exit (Log Stopped)" {
          }
          frame "Waiting for Stop", "Waiting for Stop (Log Stopped)" {
          }
          frame "Waiting for Exit (Acq Stopped)" {
            # "If we are waiting to exit, and the acquisition has already stopped, then the \"Logging Stopped\" message indicates that it is time to exit."
            n130 = call-poly "Enqueue Message.vi"("Priority Message? (F)"=TRUE, "error in (no error)"=w371, "Message"="Exit", "Message Queue"=w369) -> ("error out"=w370:errorcluster)  [unwired: 6 in, 1 out]
          }
          frame "Waiting for Stop (Acq Stopped)" {
            # "If we are waiting to stop, and the acquisition has already stopped, then the \"Logging Stopped\" message indicates that it is time to stop."
            n131 = call-poly "Enqueue Message.vi"("error in (no error)"=w377, "Message Data"="Ready..." ("Message"), "Message"="Update Status", "Message Queue"=w375) -> ("error out"=w376:errorcluster)  [unwired: 6 in, 1 out]
          }
        }
        n132 = Unbundle By Name(w352) -> ("Sonicator Module Config.Process Name"=w356:string)
        n133 = Concatenate Strings(w356, " Logging Stopped" ("text")) -> (w354:string)
        n134 = call "Write to Log File.vi"("error in"=w353, "text"=w354) -> ()  [unwired: 9 in, 1 out]
      }
      frame "Send to Sequence" {
        n135 = Variant To Data(error in=w384, type=refnum<queue> refnum ("Message Queue"), Variant=w385) -> (data=w382:refnum<queue>, error out=w383:errorcluster)
        n136 = local read "Display Cluster"() -> (w380:cluster{"User Name":string, "µm":dbl, "W":dbl})
        n137 = Unbundle By Name(w380) -> ("µm"=w379:dbl)
        n138 = call-poly "Enqueue Message.vi"("error in (no error)"=w383, "Message Data"=w379, "Message"="Sent to Sequence", "Message Queue"=w382) -> ("error out"=w387:errorcluster)  [unwired: 6 in, 1 out]
      }
      frame "Start" {
        # "Message Acquisition and Logging loops to start"
        # "Start - Enable/Disable buttons appropriately for an acquisition that has started, and update status display."
        n139 = call-poly "Enqueue Message.vi"("error in (no error)"=w397, "Message"="Start Loops", "Message Queue"=w398) -> ("error out"=w399:errorcluster)  [unwired: 7 in, 1 out]
        n140 = Merge Errors(w399) -> (w393:errorcluster)
        n141 = Unbundle By Name(w392) -> ("Sonicator Module Config.Process Name"=w396:string)
        n142 = Concatenate Strings(w396, " Start" ("text")) -> (w394:string)
        n143 = call "Write to Log File.vi"("error in"=w393, "text"=w394) -> ()  [unwired: 9 in, 1 out]
      }
      frame "Sequence Start" {
        # "Message Acquisition and Logging loops to start"
        n144 = call-poly "Enqueue Message.vi"("error in (no error)"=w403, "Message"="Broadcast settings", "Message Queue"=w402) -> ("error out"=w410:errorcluster, "dup Message Queue"=w411:refnum<queue>)  [unwired: 7 in]
        n145 = case shown="False" w404 {
          selector: w404 -> [_ w423]
          tunnel: [TRUE w423] -> w405
          tunnel: w410 -> [w421 w424]
          tunnel: w411 -> [w419 _]
          tunnel: [w418 w424] -> w415
          frame False {
            # "Start the loop if it isn't started yet"
            n146 = call-poly "Enqueue Message.vi"("error in (no error)"=w421, "Message"="Start Loops", "Message Queue"=w419) -> ("error out"=w418:errorcluster)  [unwired: 7 in, 1 out]
          }
          frame True {
          }
        }
        n147 = Bundle By Name(cluster=w409, "State"=State_Enum."Measuring") -> (w408:T7)
        n148 = Merge Errors(w415) -> (w406:errorcluster)
        n149 = Unbundle By Name(w408) -> ("Sonicator Module Config.Process Name"=w414:string)
        n150 = Concatenate Strings(w414, " Sequence Start" ("text")) -> (w412:string)
        n151 = call "Write to Log File.vi"("error in"=w406, "text"=w412) -> ()  [unwired: 9 in, 1 out]
      }
      frame "Start Loops" {
        # "I'm not sure what we would have multiple Process names in a module for but i'll leave it for now."
        # "Message Acquisition and Logging loops to start"
        # "Start - Enable/Disable buttons appropriately for an acquisition that has started, and update status display."
        n152 = Build Array(w434) -> (w432:refnum<queue>[])
        n153 = Unbundle By Name(w431) -> ("Sonicator Module Config.Process Name"=w425:string)
        n154 = for {
          tunnel: w430 -> [w439]
          tunnel: [w438] -> w433 mode=indexing
          tunnel: w432 -> [w437] mode=indexing
          tunnel: w425 -> [w436]
          n155 = call-poly "Enqueue Message.vi"("error in (no error)"=w439, "Message Data"=w436, "Message"="Start", "Message Queue"=w437) -> ("error out"=w438:errorcluster)  [unwired: 6 in, 1 out]
        }
        n156 = Merge Errors(w430, w433) -> (w427:errorcluster)
        n157 = call "Generate Temporary Report.vi"("error in (no error)"=w427, "Line of Events"=string[] ["Started"], "Module Name"=w425) -> ("error out"=w426:errorcluster)  [unwired: 8 in]
      }
      frame "Start Log" {
        # "I'm not sure what we would have multiple Process names in a module for but i'll leave it for now."
        # "Message Acquisition and Logging loops to start"
        # "Start - Enable/Disable buttons appropriately for an acquisition that has started, and update status display."
        n158 = Build Array(w451) -> (w449:refnum<queue>[])
        n159 = Unbundle By Name(w443) -> ("Sonicator Module Config.Process Name"=w448:string)
        n160 = for {
          tunnel: w442 -> [w456]
          tunnel: [w455] -> w450 mode=indexing
          tunnel: w449 -> [w454] mode=indexing
          tunnel: w448 -> [w453]
          n161 = call-poly "Enqueue Message.vi"("error in (no error)"=w456, "Message Data"=w453, "Message"="Start Log", "Message Queue"=w454) -> ("error out"=w455:errorcluster)  [unwired: 6 in, 1 out]
        }
        n162 = Merge Errors(w442, w450) -> (w444:errorcluster)
        n163 = Unbundle By Name(w443) -> ("Sonicator Module Config.Process Name"=w447:string)
        n164 = Concatenate Strings(w447, " Start Log" ("text")) -> (w445:string)
        n165 = call "Write to Log File.vi"("error in"=w444, "text"=w445) -> ()  [unwired: 9 in, 1 out]
      }
      frame "Stop" {
        # "Stop - Enable/Disable buttons appropriately for an acquisition that has stopped, and update status display."
        n166 = call-poly "Enqueue Message.vi"("error in (no error)"=w470, "Message Data"="Ready..." ("Ready..."), "Message"="Update Status", "Message Queue"=w475) -> ("error out"=w468:errorcluster)  [unwired: 6 in, 1 out]
        n167 = call-poly "Enqueue Message.vi"("error in (no error)"=w468, "Message"="Pause", "Message Queue"=w469) -> ("error out"=w466:errorcluster)  [unwired: 7 in, 1 out]
        n168 = case shown="Default" w471 {
          selector: w471 -> [_ w477]
          tunnel: [UI_State."Waiting for Stop" ("UI State") w477] -> w472
          frame Default {
          }
          frame "Waiting for Exit" {
          }
        }
        n169 = Merge Errors(w466) -> (w459:errorcluster)
        n170 = Unbundle By Name(w463) -> ("Sonicator Module Config.Process Name"=w460:string)
        n171 = call "Generate Temporary Report.vi"("error in (no error)"=w459, "Line of Events"=string[] ["Stopped"], "Module Name"=w460) -> ("error out"=w458:errorcluster)  [unwired: 8 in]
        n172 = Concatenate Strings(w460, " Stop" ("text")) -> (w464:string)
        n173 = call "Write to Log File.vi"("error in"=w458, "text"=w464) -> ()  [unwired: 9 in, 1 out]
      }
      frame "Update Status" {
        # "Update Display - Convert the message data to a string to display in the Status indicator."
        n174 = Variant To Data(error in=w485, type="", Variant=w484) -> (data=→"Status":string, error out=w482:errorcluster)
        n175 = Merge Errors(w482) -> (w486:errorcluster)
      }
      frame Default {
        # "'Default' case only runs if there is a message that isn't defined in any of the other cases.  Output a programming error."
        n176 = Concatenate Strings("The invalid message string " ("string"), w489, " was received in Scale Module Main" ("string")) -> (w490:string)
        n177 = Bundle By Name(cluster=errorcluster {"status"=TRUE, "code"=1, "source"=""} ("error constant"), "source"=w490) -> (w488:errorcluster)
        n178 = Unbundle By Name(w494) -> ("Sonicator Module Config.Process Name"=w497:string)
        n179 = Concatenate Strings(w497, "Invalid Message Recieved" ("text"), w489) -> (w495:string)
        n180 = call "Write to Log File.vi"("error in"=w488, "text"=w495) -> ()  [unwired: 9 in, 1 out]
      }
    }
    n181 = call "Error Handler - Message Handling Loop.vi"("error in (no error)"=w82, "Message Queue"=w80) -> ("dup error in"=w81:errorcluster, "dup Message Queue"=w69:refnum<queue>)  [unwired: 8 in]
  }
  n182 = while {
    tunnel: w22 -> [w511]
    tunnel: [w513] -> w28
    shift-right: [w512] -> w23
    shift-left: w26 -> [w517]
    tunnel: [w510] -> w16
    tunnel: w15 -> [w510]
    tunnel: w12 -> [w509]
    shift-right: [w506] -> _
    shift-left: w6 -> [w505]
    tunnel: [w501] -> w5
    tunnel: [w500] -> w4
    tunnel: w1 -> [w499]
    stop <- w516 stop-if-true
    # "Event Handling Loop"
    n183 = call "Dequeue Message.vi"("timeout in ms (-1)"=50, "Message Queue"=w509) -> ("error out"=w502:errorcluster, "Message Data"=w507:variant, "Message"=w508:string, "dup Message Queue"=w503:refnum<queue>)  [unwired: 6 in]
    n184 = Flush Queue(queue=w503, error in (no error)=w502) -> (queue out=w500:refnum<queue>)  [unwired: 2 out]
    n185 = case "Display Update" shown="\"Update\"" w508 {
      tunnel: w507 -> [_ w528]
      tunnel: [w518 w524] -> w506
      tunnel: w505 -> [w518 _]
      frame "False", Default {
      }
      frame "Update" {
        w526 = T13 {"Sonicator On?"=enum."Off", "Sonicator Amp Value"=0.0, "Sonicator Power Value"=0.0, "Cycle Period"=500.0}  # SC Display
        n186 = Variant To Data(type=w526, Variant=w528) -> (data=w527:T13)  [unwired: 1 in, 1 out]
        n187 = Unbundle By Name(w527) -> ("Sonicator On?"=w525:T14, "Sonicator Power Value"=w519:dbl, "Sonicator Amp Value"=w520:dbl, "Cycle Period"=w524:dbl)
        n188 = property on="User Name" class="Str"() -> ("Value"=w521:string)  [unwired: 2 in, 2 out]
        n189 = Bundle By Name(cluster=cluster{"User Name":string, "µm":dbl, "W":dbl} {"User Name"="", "µm"=0.0, "W"=0.0} ("Display Cluster"), "User Name"=w521, "W"=w519, "µm"=w520) -> (→"Display Cluster":cluster{"User Name":string, "µm":dbl, "W":dbl})
        n190 = property on="Image Ring" class="Ring (strict)"("Value"=w525) -> ()  [unwired: 2 in, 2 out]
      }
    }
    n191 = event shown="[1] Panel Resize" {
      selector: w517 -> [_ _ _ _ _ _ _]
      dyn-events: [_ _ _ _ _ _ _] -> w512
      timeout: w506 -> [_ _ _ _ _ _ _]
      tunnel: [_ _ _ TRUE ("Discard?") TRUE ("Discard?") _ _] -> w516
      tunnel: w511 -> [w529 w541 w544 w550 w556 w563 w573]
      tunnel: [_ _ w542 w555 _ w565 _] -> w514
      tunnel: [w529 w541 w543 w553 w556 w564 w573] -> w515
      tunnel: w499 -> [_ _ _ w548 _ w559 _]
      event Timeout {
        n192 = event-data() -> ()  [unwired: 1 in, 1 out]
      }
      event Panel Resize {
        n193 = local read "Original Width"() -> (w536:u32)
        n194 = event-data() -> ("NewBnds"=w537:T15)  [unwired: 1 in]
        n195 = call "Front End Resize.vi"("Starting Font"=12.0, "Area to Font Division"=1000.0, "Original Text Box Width"=60, "NewBnds"=w537, "Original Panel Width"=w536) -> ("New Text Box Width"=w532:u64, "New Font Size"=w535:dbl)  [unwired: 5 in]
        n196 = Add(x=u64 25, y=w532) -> (x+y=w531:u64)
        n197 = property on="User Name" class="Str"("Text.Width"=w531) -> ()  [unwired: 2 in, 2 out]
        n198 = property on="W" class="DigNum (strict)"("Text Width"=w532) -> ()  [unwired: 2 in, 2 out]
        n199 = property on="µm" class="DigNum (strict)"("Text Width"=w532) -> ()  [unwired: 2 in, 2 out]
        n200 = property on="W" class="DigNum (strict)"("NumText.FontSize"=w535) -> ()  [unwired: 2 in, 2 out]
        n201 = property on="µm" class="DigNum (strict)"("NumText.FontSize"=w535) -> ()  [unwired: 2 in, 2 out]
        n202 = Multiply(x=w532, y=0.4) -> (x*y=w534:dbl)
        n203 = property on="User Name" class="Str"("Text.Height"=w534) -> ()  [unwired: 2 in, 2 out]
        n204 = property on="W" class="DigNum (strict)"("Label.FontSize"=w535) -> ()  [unwired: 2 in, 2 out]
        n205 = property on="µm" class="DigNum (strict)"("Label.FontSize"=w535) -> ()  [unwired: 2 in, 2 out]
        n206 = property on="User Name" class="Str"("Text.FontSize"=w535) -> ()  [unwired: 2 in, 2 out]
      }
      event Panel Close? {
        w545 = TRUE  # Priority Message
        n207 = event-data() -> ()  [unwired: 1 in, 1 out]
        n208 = call-poly "Enqueue Message.vi"("Priority Message? (F)"=w545, "Message"="Confirm Quit", "Message Queue"=w544) -> ("error out"=w542:errorcluster, "dup Message Queue"=w543:refnum<queue>)  [unwired: 7 in]
        n209 = event-data("Discard?"=TRUE) -> ()  [unwired: 1 in, 1 out]
      }
      event "Exit": Value Change {
        w551 = TRUE  # Priority Message
        # "The UI Message Loop handles sending the Exit message to other loops."
        n210 = event-data() -> ()  [unwired: 1 in, 1 out]
        n211 = call-poly "Enqueue Message.vi"("Priority Message? (F)"=w551, "Message"="Exit", "Message Queue"=w550) -> ("error out"=w555:errorcluster, "dup Message Queue"=w553:refnum<queue>)  [unwired: 7 in]
        n212 = call "Generate Temporary Report.vi"("Line of Events"=string[] ["Exit"], "Module Name"=w548) -> ()  [unwired: 9 in, 1 out]
      }
      event User Event {
        # "The Message Handling Loop processed an \"Exit\" message, which fired this event to stop the Event Handling Loop."
        n213 = event-data() -> ()  [unwired: 1 in, 1 out]
        n214 = local write "Status"("Exit" ("Exit String")) -> ()
      }
      event "Settings Button": Mouse Down {
        # "Allow debugging during run with a ctrl click"
        n215 = event-data() -> ("PlatMods"=w562:T16)  [unwired: 1 in]
        n216 = Unbundle By Name(w562) -> ("Ctrl"=w561:bool)
        n217 = call "Generate Temporary Report.vi"("Line of Events"=string[] ["Settings Button Clicked"], "Module Name"=w559) -> ()  [unwired: 9 in, 1 out]
        n218 = case shown="False" w561 {
          tunnel: [w569 w570] -> w565
          tunnel: [w568 w571] -> w564
          tunnel: w563 -> [w567 w571]
          frame False {
            n219 = call-poly "Enqueue Message.vi"("Message"="Launch Settings Dialog", "Message Queue"=w567) -> ("error out"=w569:errorcluster, "dup Message Queue"=w568:refnum<queue>)  [unwired: 8 in]
          }
          frame True {
            n220 = property class="VI"("BDWin.Open"=TRUE ("Block Diagram Window:Open")) -> (error out=w570:errorcluster)  [unwired: 2 in, 1 out]
          }
        }
      }
      event Key Down {
        n221 = event-data() -> ("ScanCode"=→"ScanCode":i16)  [unwired: 1 in]
      }
    }
    n222 = call "Error Handler - Event Handling Loop.vi"("error in (no error)"=w514, "Message Queue"=w515) -> ("dup error in"=w513:errorcluster, "dup Message Queue"=w501:refnum<queue>)  [unwired: 8 in]
  }
  n223 = call "Main Loop.vi"("error in (no error)"=w11, "Chart Notifier"=w17, "Message Queues"=w10) -> ("error out"=w18:errorcluster)  [unwired: 8 in]
  n224 = Unregister For Events(event registration refnum=w23, error in=w28) -> (error out=w24:errorcluster)
  n225 = Merge Errors(w24, w29, w11, w18) -> (w27:errorcluster)
  n226 = Close Reference(reference=w16) -> ()  [unwired: 1 in, 1 out]
  n227 = Release Queue(queue=w4) -> ()  [unwired: 2 in, 3 out]
  n228 = Release Queue(queue=w3) -> ()  [unwired: 2 in, 3 out]
  n229 = call "Destroy User Event - Stop.vi"("error in (no error)"=w27, "User Event - Stop"=w25) -> ("error out"=w7:errorcluster)  [unwired: 9 in]
  n230 = Release Queue(queue=w5) -> ()  [unwired: 2 in, 3 out]
  n231 = flat-sequence {
    tunnel: w7 -> [_]
    frame #0 {
      n232 = invoke class="VI" method="FP.Close"() -> ()  [unwired: 3 in, 3 out]
    }
  }
